vi "VCI_InitCAN.vi"(7 "VCI_INIT_CONFIG":T1={"AccCode"=0, "AccMask"=0, "InitFlag"=0, "Fliter"=3, "Timing0"=0, "Timing1"=0, "Mode"=0} {"Fliter" items=["接收所有类型"=3, "只接收标准帧"=4, "只接收扩展帧"=7]; "Mode" items=["正常工作", "自测模式（环回）", "仅侦听模式"]; "InitFlag" items=["使用Flash参数", "使用界面设置参数"]}, 8 "error in (no error)":errorcluster caption="错误输入（无错误）", 9 "CANIndex":u32, 10 "DevIndex":u32, 11 "DevType":T5=2 items=["USB-CAN"=2, "USB-CAN2"=3]) -> (0 "error out":errorcluster caption="错误输出", 3 "Return Val":T6=1 items=["OK"=1, "ERROR1"=0, "ERROR2"=-1])   [LabVIEW 2018, in "ControlCan.lvlib"]
uses:
  ControlCan.lvlib
  Return Val.ctl
  DevType.ctl
  VCI_INIT_CONFIG.ctl
  InitFlag.ctl
  Fliter.ctl
  Mode.ctl
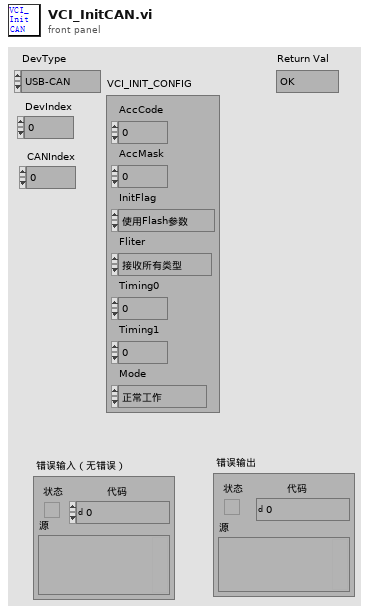
[diagram p1: front panel]
types:
  T1 = typedef "ControlCAN.lvlib/VCI_INIT_CONFIG.ctl" = cluster{"AccCode":u32, "AccMask":u32, "InitFlag":T2, "Fliter":T3, "Timing0":u8, "Timing1":u8, "Mode":T4}
  T2 = typedef "ControlCAN.lvlib/InitFlag.ctl" = u32
  T3 = typedef "ControlCAN.lvlib/Fliter.ctl" = u8
  T4 = typedef "ControlCAN.lvlib/Mode.ctl" = u8
  T5 = typedef "ControlCAN.lvlib/DevType.ctl" = u32
  T6 = typedef "ControlCAN.lvlib/Return Val.ctl" = i32
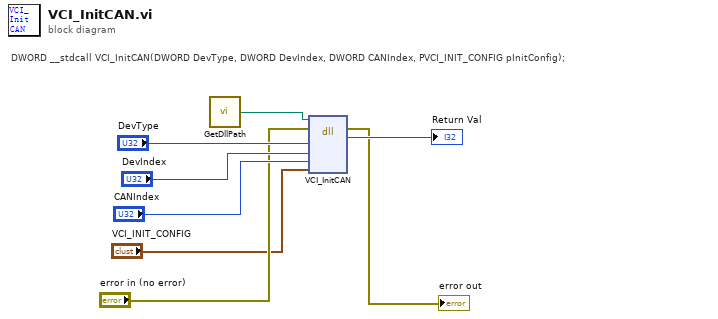
[diagram p0: block diagram]
diagram:
  # "DWORD __stdcall VCI_InitCAN(DWORD DevType, DWORD DevIndex, DWORD CANIndex, PVCI_INIT_CONFIG pInitConfig);"
  n1 = call "GetDllPath.vi"() -> ("DllPath"=w1:path)  [unwired: 1 out]
  n2 = dll-call lib="?" fn="VCI_InitCAN"(path in=w1, error in="error in (no error)", "DevType"="DevType", "DevIndex"="DevIndex", "CANIndex"="CANIndex", "pInitConfig"="VCI_INIT_CONFIG") -> (error out=→"error out":errorcluster, "ReturnVal"=→"Return Val":i32)  [unwired: 5 in, 1 out]
